vi "Pressure Queue Consumer Loop.vi"(0 "Save File Connection X":refnum<vi>, 1 "Start Time Reactor X":refnum<vi>, 2 "Queue Reactor X":refnum<vi>, 3 "Current Cycle Reactor X":refnum<vi>, 4 "Save File JSON Connection X":refnum<vi>, 5 "Logging Data X":refnum<vi>, 6 "Reactor Name":string, 9 "Reactor Number":i32, 11 "Stop Program":refnum<vi>) -> ()   [LabVIEW 2021]
uses:
  <vilib>/Utility/error.llb/DialogType.ctl
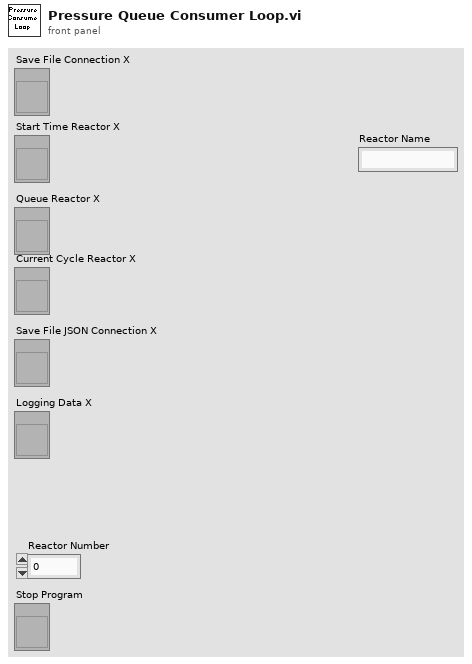
[diagram p1: front panel]
types:
  T1 = enum16{" 0 - write pressure", "1 - close then reopen file on google drive ", "2 - close reopened file on google drive open file on local drive", "3 - close file on local drive and stop"}
  T2 = cluster{"type":string, "meta":string, "payload":string}
  T3 = cluster{"TimeElapsed":string, "CurrentCycle":string, "Pressure":string, "GUID":string}
  T4 = typedef "DialogType.ctl" = u16
  T5 = enum16{"open", "replace", "create", "open or create", "replace or create", "replace or create with confirmation"}
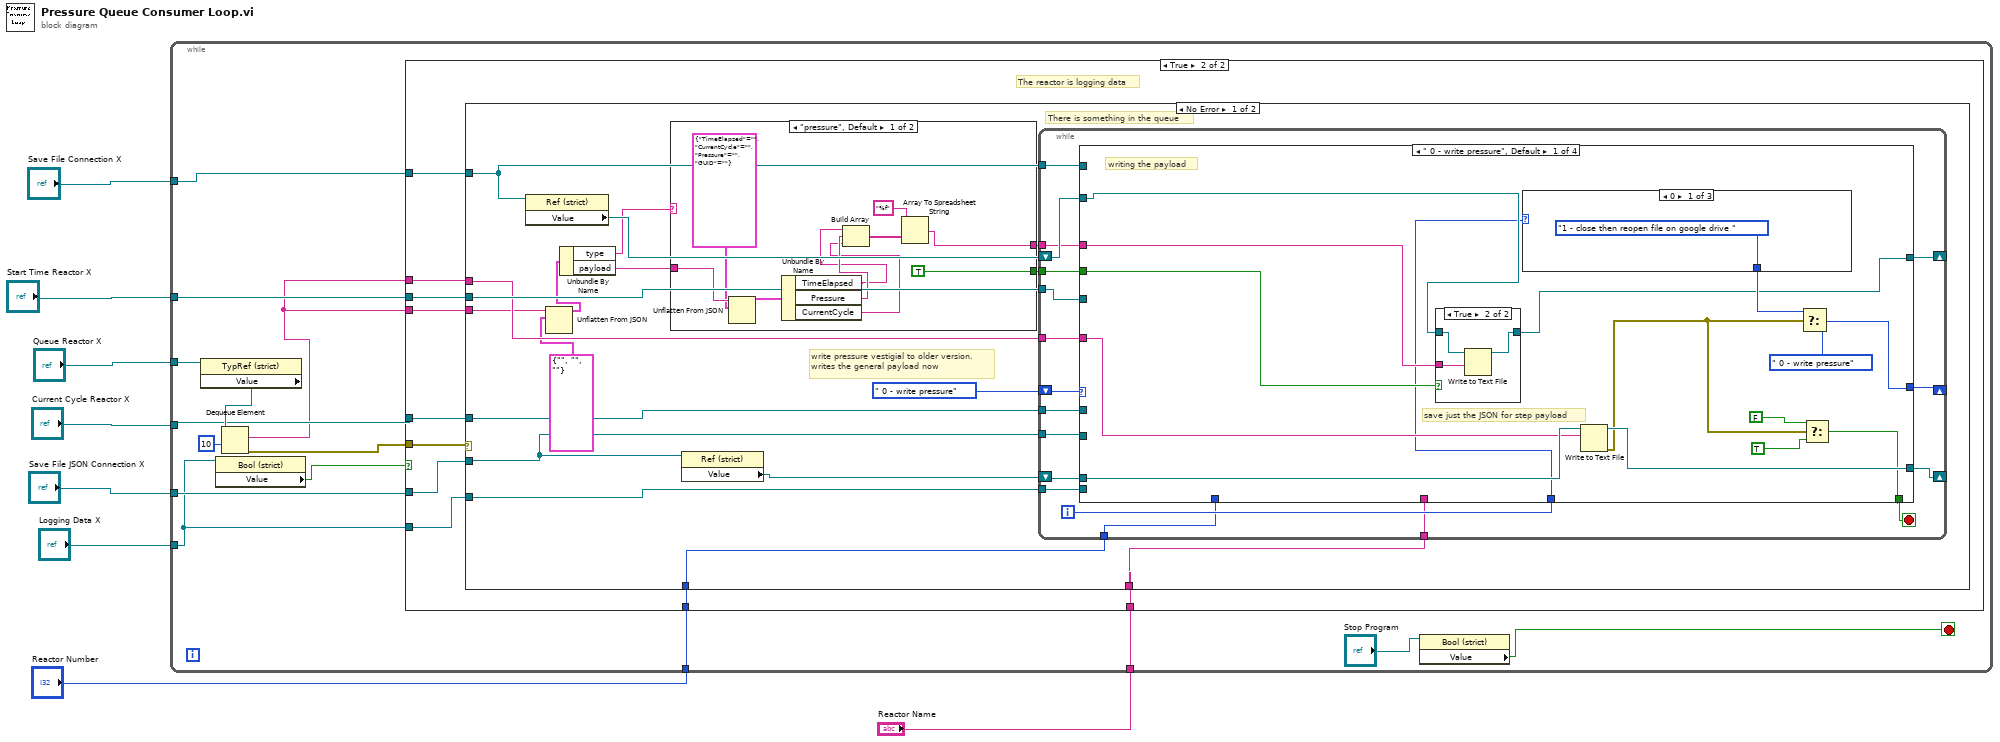
[diagram p0: block diagram]
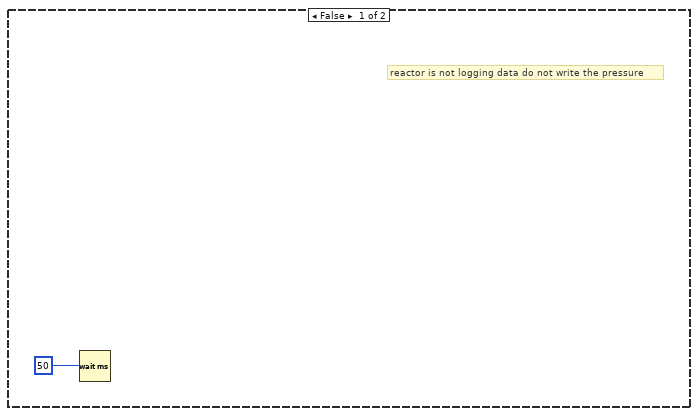
[diagram p2: hidden frame]
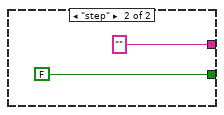
[diagram p3: hidden frame]
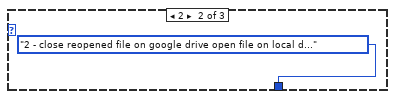
[diagram p5: hidden frame]
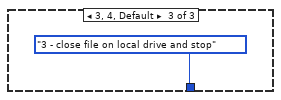
[diagram p6: hidden frame]
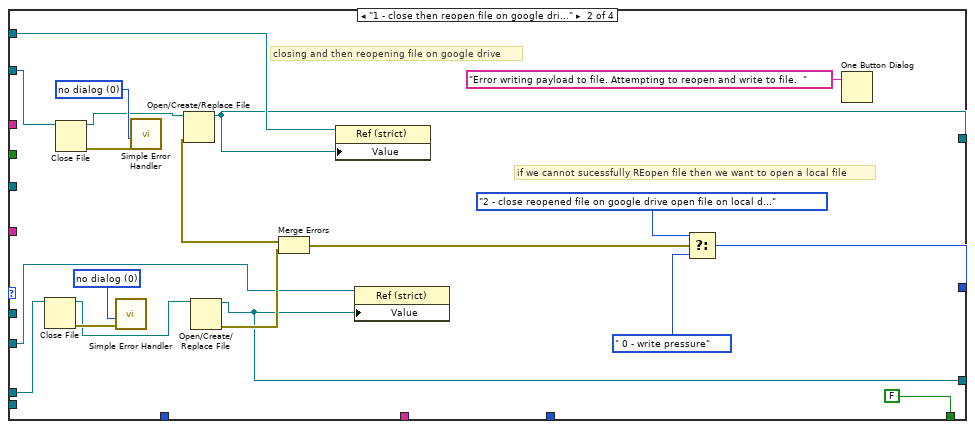
[diagram p7: hidden frame]
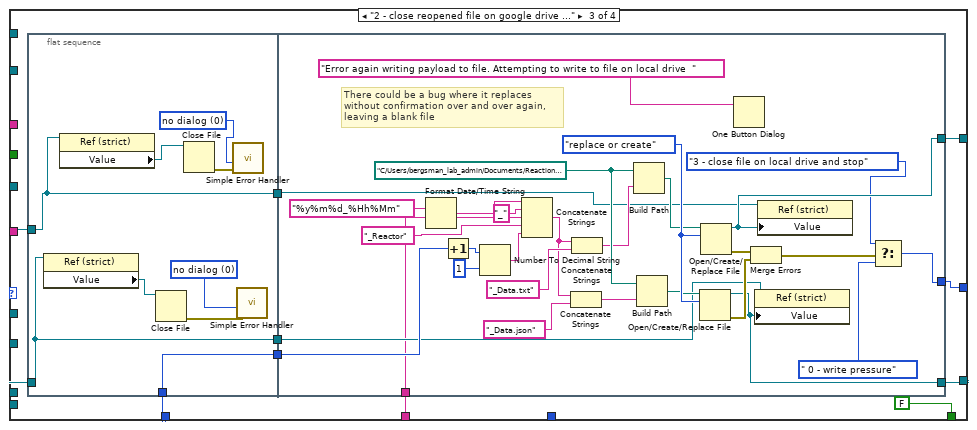
[diagram p8: hidden frame]
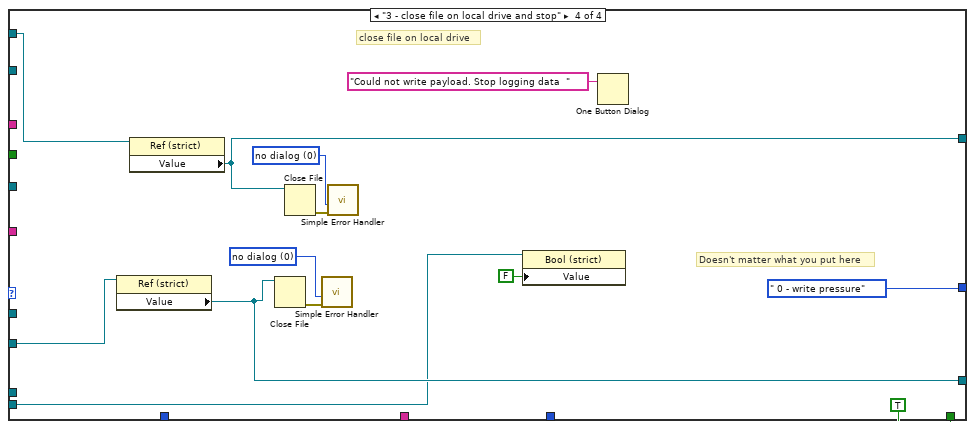
[diagram p9: hidden frame]
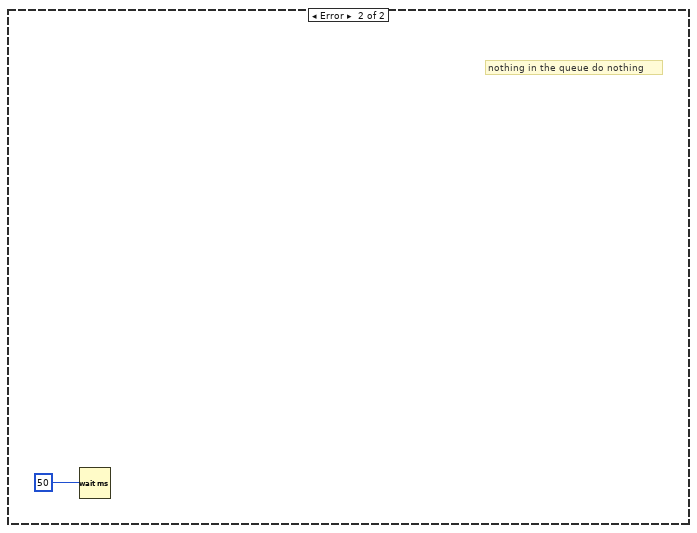
[diagram p10: hidden frame]
diagram:
  n1 = while {
    tunnel: "Logging Data X" -> [w17]
    tunnel: "Queue Reactor X" -> [w22]
    tunnel: "Start Time Reactor X" -> [w21]
    tunnel: "Current Cycle Reactor X" -> [w20]
    tunnel: "Save File JSON Connection X" -> [w19]
    tunnel: "Save File Connection X" -> [w18]
    tunnel: "Reactor Number" -> [w14]
    tunnel: "Reactor Name" -> [w10]
    stop <- w12 stop-if-true
    n2 = property class="TypRef (strict)"(reference=w22) -> ("Value"=w23:refnum<queue>)  [unwired: 1 in, 2 out]
    n3 = property class="Bool (strict)"(reference=w17) -> ("Value"=w15:bool)  [unwired: 1 in, 2 out]
    n4 = Dequeue Element(queue=w23, timeout in ms (-1)=10) -> (element=w9:string, error out=w16:errorcluster)  [unwired: 1 in, 2 out]
    n5 = case shown="True" w15 {
      tunnel: w21 -> [_ w34]
      tunnel: w20 -> [_ w33]
      tunnel: w9 -> [_ w32]
      tunnel: w19 -> [_ w31]
      tunnel: w18 -> [_ w30]
      tunnel: w17 -> [_ w29]
      tunnel: w16 -> [_ w28]
      tunnel: w14 -> [_ w27]
      tunnel: w10 -> [_ w26]
      tunnel: w9 -> [_ w25]
      frame False {
        # "reactor is not logging data do not write the pressure"
        n6 = Wait (ms)(milliseconds to wait=u32 50 ("millisecond multiple")) -> ()  [unwired: 1 out]
      }
      frame True {
        # "The reactor is logging data"
        n7 = case shown="No Error" w28 {
          tunnel: w34 -> [w52 _]
          tunnel: w33 -> [w51 _]
          tunnel: w32 -> [w43 _]
          tunnel: w31 -> [w46 _]
          tunnel: w30 -> [w47 _]
          tunnel: w29 -> [w48 _]
          tunnel: w27 -> [w45 _]
          tunnel: w26 -> [w44 _]
          tunnel: w25 -> [w41 _]
          frame No Error {
            # "write pressure vestigial to older version. writes the general payload now"
            # "There is something in the queue"
            n8 = property class="Ref (strict)"(reference=w47) -> ("Value"=w50:refnum<file>)  [unwired: 1 in, 2 out]
            n9 = Unflatten From JSON(JSON string=w41, type and defaults=T2 {"type"="", "meta"="", "payload"=""} ("input cluster")) -> (value=w40:T2)  [unwired: 5 in, 1 out]
            n10 = Unbundle By Name(w40) -> ("type"=w36:string, "payload"=w38:string)
            n11 = case shown="\"pressure\", Default" w36 {
              tunnel: w38 -> [w62 _]
              tunnel: [w56 "" ("spreadsheet string")] -> w37
              tunnel: [TRUE FALSE] -> w35
              frame "pressure", Default {
                n12 = Unflatten From JSON(JSON string=w62, type and defaults=T3 {"TimeElapsed"="", "CurrentCycle"="", "Pressure"="", "GUID"=""} ("input cluster")) -> (value=w60:T3)  [unwired: 5 in, 1 out]
                n13 = Unbundle By Name(w60) -> ("TimeElapsed"=w55:string, "Pressure"=w57:string, "CurrentCycle"=w54:string)
                n14 = Build Array(w55, w57, w54) -> (w58:string[])
                n15 = Array To Spreadsheet String(array=w58, 3:"%f" ("format string")) -> (spreadsheet string=w56:string)  [unwired: 1 in]
              }
              frame "step" {
              }
            }
            n16 = property class="Ref (strict)"(reference=w46) -> ("Value"=w49:refnum<file>)  [unwired: 1 in, 2 out]
            n17 = while {
              shift-right: [w76] -> _
              shift-left: T1." 0 - write pressure" -> [w70]
              tunnel: w52 -> [w81]
              tunnel: w51 -> [w80]
              shift-right: [w78] -> _
              shift-left: w50 -> [w82]
              shift-right: [w77] -> _
              shift-left: w49 -> [w79]
              tunnel: w48 -> [w75]
              tunnel: w47 -> [w72]
              tunnel: w46 -> [w71]
              tunnel: w45 -> [w69]
              tunnel: w44 -> [w68]
              tunnel: w43 -> [w67]
              tunnel: w37 -> [w66]
              tunnel: w35 -> [w65]
              i -> [w73]
              stop <- w74 stop-if-true
              n18 = case shown="\" 0 - write pressure\", Default" w70 {
                tunnel: w82 -> [w87 w120 _ _]
                tunnel: w81 -> [_ _ _ _]
                tunnel: w80 -> [_ _ _ _]
                tunnel: w79 -> [w97 w119 _ _]
                tunnel: [w88 w106 w134 w181] -> w78
                tunnel: [w96 w113 w133 w180] -> w77
                tunnel: [w95 w108 w132 T1." 0 - write pressure"] -> w76
                tunnel: w75 -> [_ _ _ w178]
                tunnel: [w93 FALSE FALSE TRUE] -> w74
                tunnel: w73 -> [w83 _ _ _]
                tunnel: w72 -> [_ w112 w131 w175]
                tunnel: w71 -> [_ w111 w130 w174]
                tunnel: w69 -> [_ _ w126 _]
                tunnel: w68 -> [_ _ w125 _]
                tunnel: w67 -> [w86 _ _ _]
                tunnel: w66 -> [w85 _ _ _]
                tunnel: w65 -> [w84 _ _ _]
                frame " 0 - write pressure", Default {
                  # "save just the JSON for step payload"
                  # "writing the payload"
                  n19 = case shown="True" w84 {
                    tunnel: [w98 w101] -> w88
                    tunnel: w87 -> [w98 w100]
                    tunnel: w85 -> [_ w99]
                    frame False {
                    }
                    frame True {
                      n20 = Write to Text File(file (use dialog)=w100, text=w99) -> (refnum out=w101:refnum<file>)  [unwired: 2 in, 2 out]
                    }
                  }
                  n21 = case shown="0" w83 {
                    tunnel: [T1."1 - close then reopen file on google drive " T1."2 - close reopened file on google drive open file on local drive" T1."3 - close file on local drive and stop"] -> w89
                    frame 0 {
                    }
                    frame 2 {
                    }
                    frame 3, 4, Default {
                    }
                  }
                  n22 = Write to Text File(file (use dialog)=w97, text=w86) -> (refnum out=w96:refnum<file>, error out=w90:errorcluster)  [unwired: 2 in, 1 out]
                  n23 = Select(t=w89, s=w90, f=T1." 0 - write pressure") -> (s? t:f=w95:T1)
                  n24 = Select(t=FALSE, s=w90, f=TRUE) -> (s? t:f=w93:bool)
                }
                frame "1 - close then reopen file on google drive " {
                  w121 = T4 0 items=["no dialog", "OK message", "continue or stop message", "OK message + warnings", "continue/stop + warnings"] ("type of dialog (OK msg:1)")
                  w124 = T4 0 items=["no dialog", "OK message", "continue or stop message", "OK message + warnings", "continue/stop + warnings"] ("type of dialog (OK msg:1)")
                  # "closing and then reopening file on google drive"
                  # "if we cannot sucessfully REopen file then we want to open a local file"
                  n25 = Close File(refnum=w119) -> (path=w118:path, error out=w122:errorcluster)  [unwired: 1 in]
                  n26 = Close File(refnum=w120) -> (path=w117:path, error out=w123:errorcluster)  [unwired: 1 in]
                  n27 = call <vilib>:"Simple Error Handler.vi"("type of dialog (OK msg:1)"=w121, "error in (no error)"=w122) -> ()  [unwired: 3 in, 5 out]
                  n28 = call <vilib>:"Simple Error Handler.vi"("type of dialog (OK msg:1)"=w124, "error in (no error)"=w123) -> ()  [unwired: 3 in, 5 out]
                  n29 = Open/Create/Replace File(file path (use dialog)=w117) -> (refnum out=w106:refnum<file>, error out=w115:errorcluster)  [unwired: 5 in, 1 out]
                  n30 = Open/Create/Replace File(file path (use dialog)=w118) -> (refnum out=w113:refnum<file>, error out=w116:errorcluster)  [unwired: 5 in, 1 out]
                  n31 = Merge Errors(w115, w116) -> (w105:errorcluster)
                  n32 = property class="Ref (strict)"(reference=w112, "Value"=w106) -> ()  [unwired: 1 in, 2 out]
                  n33 = property class="Ref (strict)"(reference=w111, "Value"=w113) -> ()  [unwired: 1 in, 2 out]
                  n34 = Select(t=T1."2 - close reopened file on google drive open file on local drive", s=w105, f=T1." 0 - write pressure") -> (s? t:f=w108:T1)
                  n35 = One Button Dialog(message="Error writing payload to file. Attempting to reopen and write to file.  ") -> ()  [unwired: 1 in, 1 out]
                }
                frame "2 - close reopened file on google drive open file on local drive" {
                  n36 = flat-sequence {
                    tunnel: w130 -> [w137]
                    tunnel: w131 -> [w138]
                    tunnel: [w136] -> w129
                    tunnel: [w138] -> w128
                    tunnel: [w137] -> w127
                    tunnel: w126 -> [w136]
                    tunnel: [w170] -> w134
                    tunnel: [w169] -> w133
                    tunnel: [w166] -> w132
                    tunnel: w129 -> [w156]
                    tunnel: w128 -> [w150]
                    tunnel: w127 -> [w149]
                    tunnel: w125 -> [w145]
                    frame #0 {
                      w139 = T4 0 items=["no dialog", "OK message", "continue or stop message", "OK message + warnings", "continue/stop + warnings"] ("type of dialog (OK msg:1)")
                      w142 = T4 0 items=["no dialog", "OK message", "continue or stop message", "OK message + warnings", "continue/stop + warnings"] ("type of dialog (OK msg:1)")
                      n37 = property class="Ref (strict)"(reference=w137) -> ("Value"=w140:refnum<file>)  [unwired: 1 in, 2 out]
                      n38 = property class="Ref (strict)"(reference=w138) -> ("Value"=w143:refnum<file>)  [unwired: 1 in, 2 out]
                      n39 = Close File(refnum=w140) -> (error out=w141:errorcluster)  [unwired: 1 in, 1 out]
                      n40 = Close File(refnum=w143) -> (error out=w144:errorcluster)  [unwired: 1 in, 1 out]
                      n41 = call <vilib>:"Simple Error Handler.vi"("type of dialog (OK msg:1)"=w142, "error in (no error)"=w144) -> ()  [unwired: 3 in, 5 out]
                      n42 = call <vilib>:"Simple Error Handler.vi"("type of dialog (OK msg:1)"=w139, "error in (no error)"=w141) -> ()  [unwired: 3 in, 5 out]
                    }
                    frame #1 {
                      w173 = T5."replace or create" ("operation (0:open)")
                      w164 = path "C:/Users/bergsman_lab_admin/Documents/Reaction_data" ("file path (use dialog)")
                      # "There could be a bug where it replaces\nwithout confirmation over and over again,\nleaving a blank file"
                      n43 = Format Date/Time String(time format string (%c)="%y%m%d_%Hh%Mm") -> (date/time string=w147:string)  [unwired: 2 in]
                      n44 = Increment(x=w156) -> (x+1=w159:i32)
                      n45 = Number To Decimal String(number=w159, width (-)=i16 1) -> (decimal integer string=w160:string)
                      n46 = Concatenate Strings(w147, "_" ("string"), w145, "_Reactor" ("string"), w160) -> (w155:string)
                      n47 = Concatenate Strings(w155, "_Data.json" ("string")) -> (w153:string)
                      n48 = Concatenate Strings(w155, "_Data.txt" ("string")) -> (w154:string)
                      n49 = Build Path(base path=w164, name or relative path=w154) -> (appended path=w152:path)
                      n50 = Build Path(base path=w164, name or relative path=w153) -> (appended path=w151:path)
                      n51 = Open/Create/Replace File(file path (use dialog)=w151, operation (0:open)=w173) -> (refnum out=w169:refnum<file>, error out=w172:errorcluster)  [unwired: 4 in, 1 out]
                      n52 = Open/Create/Replace File(file path (use dialog)=w152, operation (0:open)=w173) -> (refnum out=w170:refnum<file>, error out=w171:errorcluster)  [unwired: 4 in, 1 out]
                      n53 = One Button Dialog(message="Error again writing payload to file. Attempting to write to file on local drive  ") -> ()  [unwired: 1 in, 1 out]
                      n54 = Merge Errors(w171, w172) -> (w148:errorcluster)
                      n55 = property class="Ref (strict)"(reference=w149, "Value"=w169) -> ()  [unwired: 1 in, 2 out]
                      n56 = property class="Ref (strict)"(reference=w150, "Value"=w170) -> ()  [unwired: 1 in, 2 out]
                      n57 = Select(t=T1."3 - close file on local drive and stop", s=w148, f=T1." 0 - write pressure") -> (s? t:f=w166:T1)
                    }
                  }
                }
                frame "3 - close file on local drive and stop" {
                  w185 = T4 0 items=["no dialog", "OK message", "continue or stop message", "OK message + warnings", "continue/stop + warnings"] ("type of dialog (OK msg:1)")
                  w186 = T4 0 items=["no dialog", "OK message", "continue or stop message", "OK message + warnings", "continue/stop + warnings"] ("type of dialog (OK msg:1)")
                  # "Doesn't matter what you put here"
                  # "close file on local drive"
                  n58 = property class="Ref (strict)"(reference=w174) -> ("Value"=w180:refnum<file>)  [unwired: 1 in, 2 out]
                  n59 = property class="Ref (strict)"(reference=w175) -> ("Value"=w181:refnum<file>)  [unwired: 1 in, 2 out]
                  n60 = Close File(refnum=w180) -> (error out=w184:errorcluster)  [unwired: 1 in, 1 out]
                  n61 = Close File(refnum=w181) -> (error out=w183:errorcluster)  [unwired: 1 in, 1 out]
                  n62 = call <vilib>:"Simple Error Handler.vi"("type of dialog (OK msg:1)"=w185, "error in (no error)"=w184) -> ()  [unwired: 3 in, 5 out]
                  n63 = call <vilib>:"Simple Error Handler.vi"("type of dialog (OK msg:1)"=w186, "error in (no error)"=w183) -> ()  [unwired: 3 in, 5 out]
                  n64 = property class="Bool (strict)"(reference=w178, "Value"=FALSE) -> ()  [unwired: 1 in, 2 out]
                  n65 = One Button Dialog(message="Could not write payload. Stop logging data  ") -> ()  [unwired: 1 in, 1 out]
                }
              }
            }
          }
          frame Error {
            # "nothing in the queue do nothing"
            n66 = Wait (ms)(milliseconds to wait=u32 50 ("millisecond multiple")) -> ()  [unwired: 1 out]
          }
        }
      }
    }
    n67 = property class="Bool (strict)"(reference="Stop Program") -> ("Value"=w12:bool)  [unwired: 1 in, 2 out]
  }
